vi "m1m3_getEvent_HardpointMonitorInfo.vi"(8 "error in (no error)":errorcluster, 11 "logevent_HardpointMonitorInfo_Ctl":T1) -> (0 "error out":errorcluster, 2 "function return":i32, 3 "logevent_HardpointMonitorInfo_Ctl out":T1)   [LabVIEW 2016, in "SALLV_m1m3.lvlib"]
doc: "int m1m3_shm_getEvent_HardpointMonitorInfoLV(m1m3_logevent_HardpointMonitorInfoLV *logevent_HardpointMonitorInfo_Ctl );"
uses:
  SALLV_m1m3.lvlib
  DataTypes/logevent_HardpointMonitorInfo.ctl
  SALLV_m1m3.so
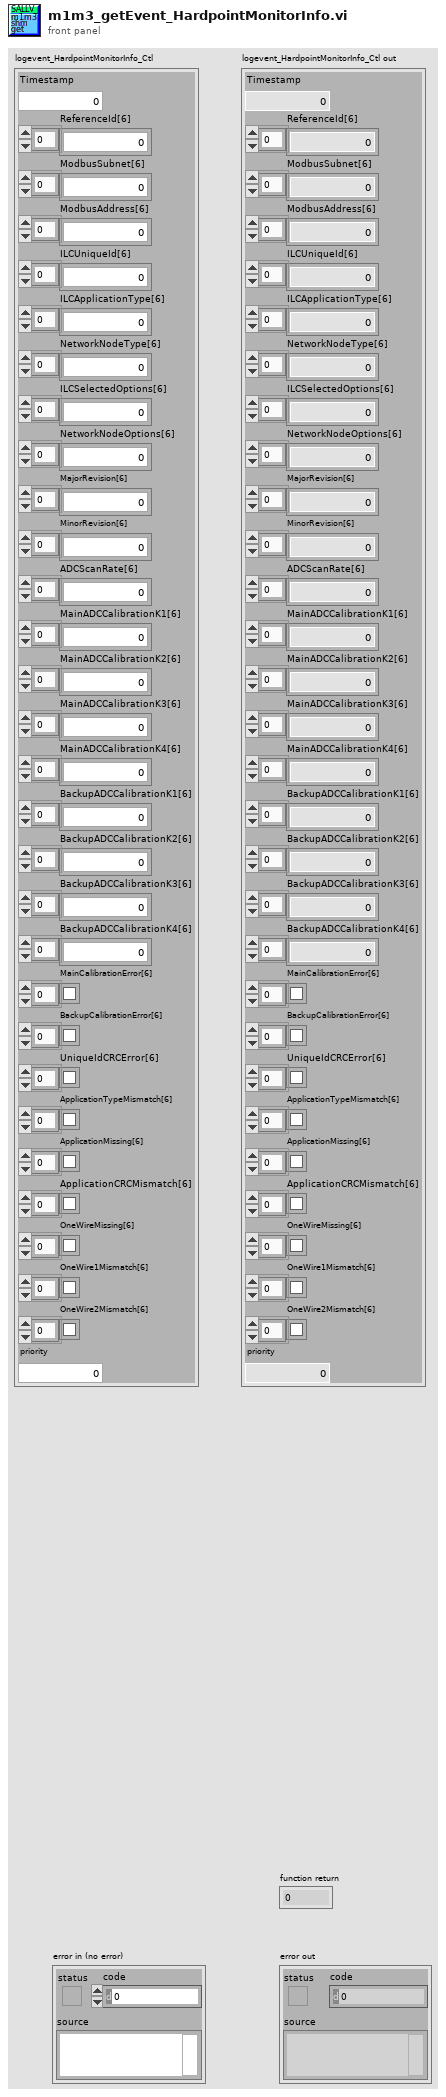
[diagram p1: front panel]
types:
  T1 = typedef "SALLV_m1m3.lvlib/logevent_HardpointMonitorInfo.ctl" = cluster{"Timestamp":dbl, "ReferenceId[6]":i32[], "ModbusSubnet[6]":u8[], "ModbusAddress[6]":u8[], "ILCUniqueId[6]":i64[], "ILCApplicationType[6]":u8[], "NetworkNodeType[6]":u8[], "ILCSelectedOptions[6]":u8[], "NetworkNodeOptions[6]":u8[], "MajorRevision[6]":u8[], "MinorRevision[6]":u8[], "ADCScanRate[6]":u8[], "MainADCCalibrationK1[6]":sgl[], "MainADCCalibrationK2[6]":sgl[], "MainADCCalibrationK3[6]":sgl[], "MainADCCalibrationK4[6]":sgl[], "BackupADCCalibrationK1[6]":sgl[], "BackupADCCalibrationK2[6]":sgl[], "BackupADCCalibrationK3[6]":sgl[], "BackupADCCalibrationK4[6]":sgl[], "MainCalibrationError[6]":bool[], "BackupCalibrationError[6]":bool[], "UniqueIdCRCError[6]":bool[], "ApplicationTypeMismatch[6]":bool[], "ApplicationMissing[6]":bool[], "ApplicationCRCMismatch[6]":bool[], "OneWireMissing[6]":bool[], "OneWire1Mismatch[6]":bool[], "OneWire2Mismatch[6]":bool[], "priority":i32}
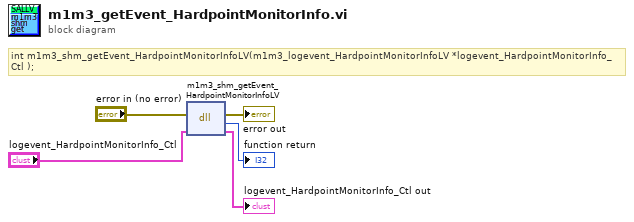
[diagram p0: block diagram]
diagram:
  # "int m1m3_shm_getEvent_HardpointMonitorInfoLV(m1m3_logevent_HardpointMonitorInfoLV *logevent_HardpointMonitorInfo_Ctl );"
  n1 = dll-call lib="opt/CODE/ts_m1m3supporteui/SALLV_m1m3/SALLV_m1m3.*" fn="m1m3_shm_getEvent_HardpointMonitorInfoLV"(error in="error in (no error)", "logevent_HardpointMonitorInfo_Ctl"="logevent_HardpointMonitorInfo_Ctl") -> (error out=→"error out":errorcluster, →"function return":i32, "logevent_HardpointMonitorInfo_Ctl"=→"logevent_HardpointMonitorInfo_Ctl out":T1)  [unwired: 2 in, 1 out]
